vi "checkROIStart.vi"(10 "lastClickPosition":cluster{"X":i32, "Y":i32}, 11 "FTTDataClusterIn":T1) -> (2 "coords":cluster{"X":i32, "Y":i32}, 3 "FTTDataClusterOut":T1)   [LabVIEW 2016]
doc: "Determine ROI start position based on specified dimension and clicked position."
uses:
  controls/UI Data.ctl
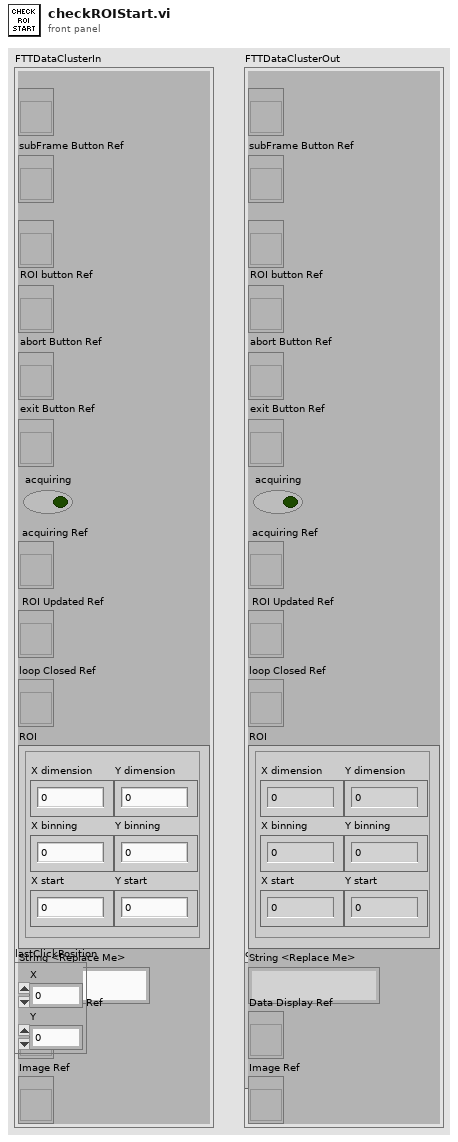
[diagram p1: front panel]
types:
  T1 = typedef "UI Data.ctl" = cluster{"full Frame Button Ref":refnum<vi>, "subFrame Button Ref":refnum<vi>, "closed Loop Button Ref":refnum<vi>, "ROI button Ref":refnum<vi>, "abort Button Ref":refnum<vi>, "exit Button Ref":refnum<vi>, "acquiring":bool, " acquiring Ref":refnum<vi>, " ROI Updated Ref":refnum<vi>, "loop Closed Ref":refnum<vi>, "ROI":cluster{"X dimension":i16, "Y dimension":i16, "X binning":i16, "Y binning":i16, "X start":i16, "Y start":i16}, "String <Replace Me>":string, "Data Display Ref":refnum<vi>, "Image Ref":refnum<vi>}
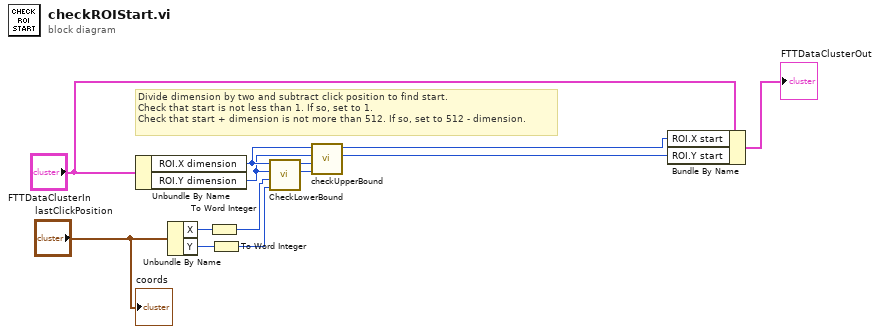
[diagram p0: block diagram]
diagram:
  # "Divide dimension by two and subtract click position to find start.\nCheck that start is not less than 1. If so, set to 1.\nCheck that start + dimension is not more than 512. If so, set to 512 - dimension."
  n1 = Unbundle By Name("FTTDataClusterIn") -> ("ROI.X dimension"=w7:i16, "ROI.Y dimension"=w6:i16)
  n2 = Unbundle By Name("lastClickPosition") -> ("X"=w4:i32, "Y"=w1:i32)
  n3 = To Word Integer(number=w4) -> (16bit integer=w3:i16)
  n4 = To Word Integer(number=w1) -> (16bit integer=w2:i16)
  n5 = call "CheckLowerBound.vi"("yClick"=w2, "xClick"=w3, "yDimension"=w6, "xDimension"=w7) -> ("yStart"=w5:i16, "xStart"=w10:i16)  [unwired: 6 in]
  n6 = call "checkUpperBound.vi"("yStart in"=w5, "xStart in"=w10, "Y dimension"=w6, "X dimension"=w7) -> ("yStart out"=w8:i16, "xStart out"=w9:i16)  [unwired: 6 in]
  n7 = Bundle By Name(cluster="FTTDataClusterIn", "ROI.X start"=w9, "ROI.Y start"=w8) -> (→"FTTDataClusterOut":T1)
  "coords" <- "lastClickPosition"
